vi "MEASURE_hysteresis_multiple_gate_Raman_single 2450 - set voltage - revised for Philipp.vi"() -> ()   [LabVIEW 2016]
uses:
  C/Program Files/National Instruments/LabVIEW 2016/instr.lib/Keithley 2450/Keithley 2450.lvlib
panel:
  out "top gate voltage":dbl format="%#_13g"
  out "loop run":i32=2
  out "top gate leaking":string="-9.306248E-12\n"
  out "while loop":dbl
  in  "Gate sequence":dbl
  in  "GATE final Value":dbl=6.0
  in  "topgate-off set":dbl=-5.0
  in  "0ff set{T}/no off set[F]":bool
  in  "loop #":i32=2
  in  "GATE STEP(mv)":i32=100
  in  "GATE Low Value (default 0)":dbl
  in  "GATE High Value":dbl=6.0
  in  "Function (0: Volts) 2":u16(ring) items=["Volts", "Current", "Resistance"]
  in  "Source Compaliance":dbl=1.000000000000001e-07
  in  "topgate address":refnum<visa-resource-name>="GPIB0::20::INSTR"
  in  "GATE / SD stablization 3":dbl=0.2 format="%#_13g"
  # "Gate 2450 Setting"
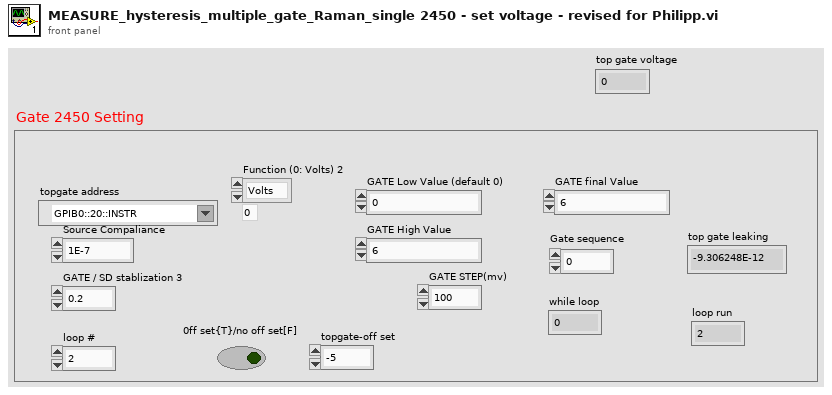
[diagram p1: front panel]
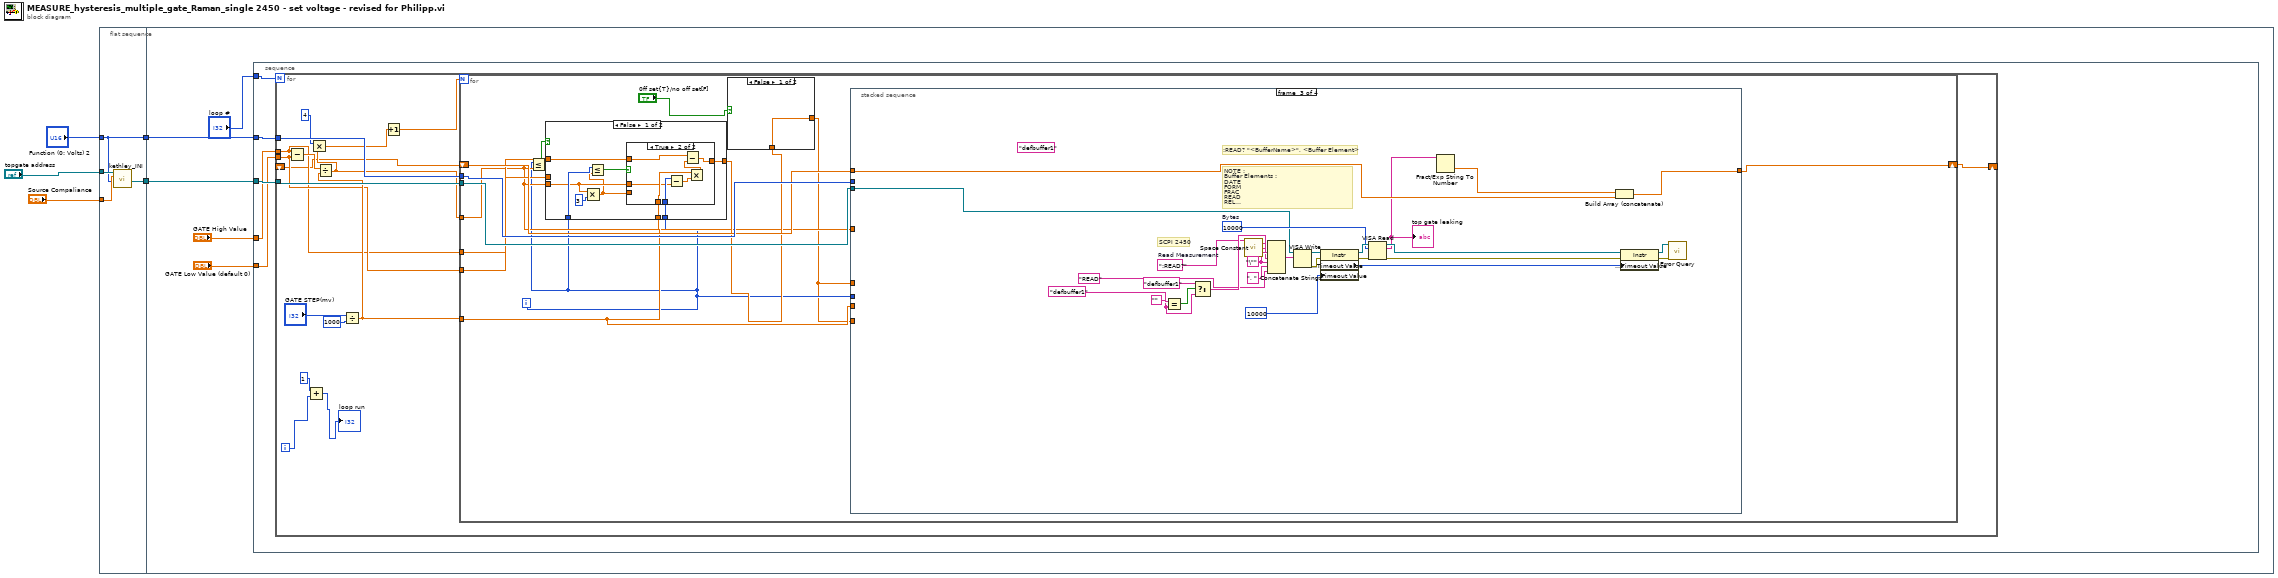
[diagram p0: block diagram]
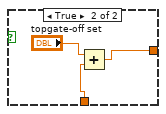
[diagram p2: hidden frame]
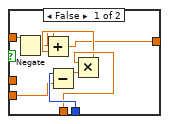
[diagram p3: hidden frame]
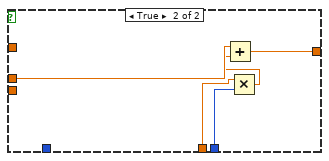
[diagram p4: hidden frame]
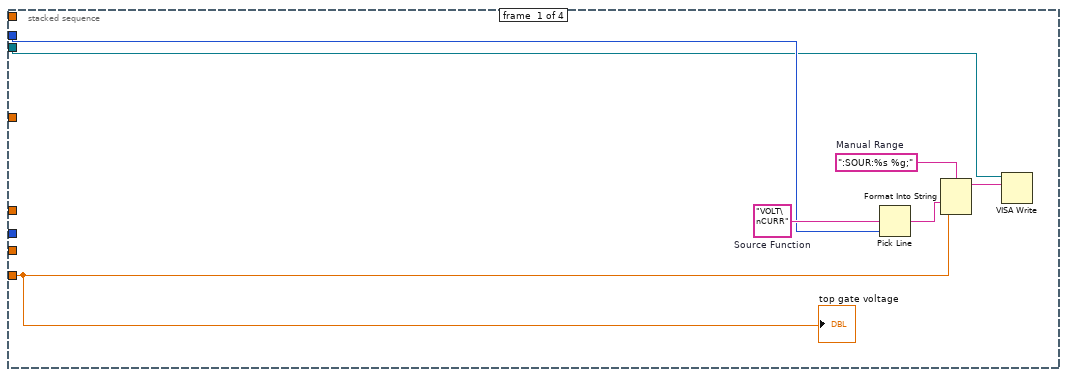
[diagram p5: hidden frame]
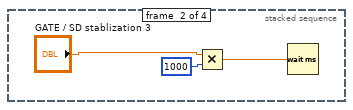
[diagram p6: hidden frame]
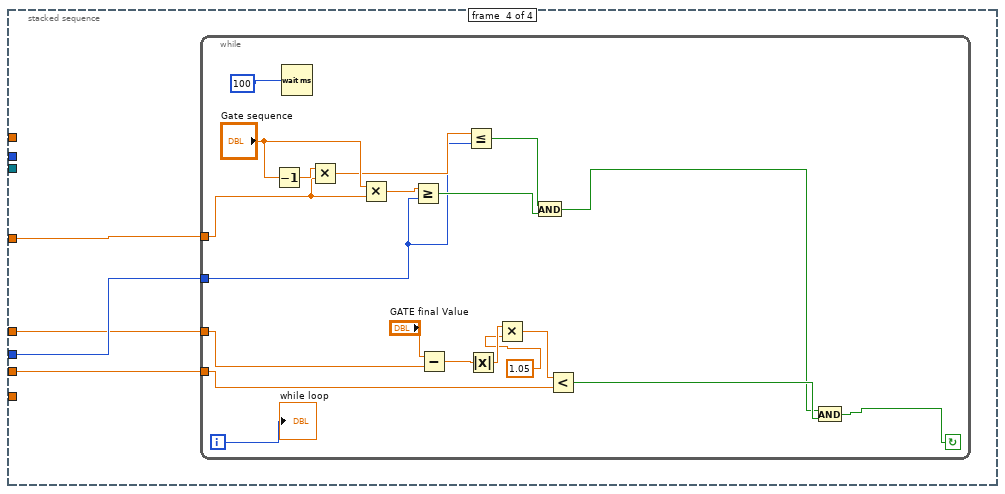
[diagram p7: hidden frame]
diagram:
  n1 = flat-sequence {
    tunnel: "topgate address" -> [w9]
    tunnel: "Source Compaliance" -> [w8]
    tunnel: "Function (0: Volts) 2" -> [w6]
    tunnel: [w7] -> w2
    tunnel: [w6] -> w1
    tunnel: w2 -> [w14]
    tunnel: w1 -> [w13]
    frame #0 {
      n2 = call "kethley_INI.vi"("Function (0: Volts) in"=w6, "Source Compaliance"=w8, "VISA Refnum in"=w9) -> ("VISA resource name out"=w7:refnum<visa-resource-name>)  [unwired: 8 in]
    }
    frame #1 {
      n3 = stacked-sequence {
        tunnel: w14 -> [w18]
        tunnel: w13 -> [w19]
        tunnel: "GATE High Value" -> [w16]
        tunnel: "GATE Low Value (default 0)" -> [w17]
        tunnel: "loop #" -> [w15]
        frame #0 {
          n4 = for {
            N: w15 -> [_]
            tunnel: w19 -> [w36]
            tunnel: w18 -> [w35]
            tunnel: w17 -> [w29]
            tunnel: w16 -> [w28]
            shift-right: [w24] -> _
            shift-left: _ -> [w23]
            i -> [w21]
            n5 = Subtract(x=w28, y=w29) -> (x-y=w31:dbl)
            n6 = Add(x=1, y=w21) -> (x+y=→"loop run":i32)
            n7 = Divide(x="GATE STEP(mv)", y=1000) -> (x/y=w30:dbl)
            n8 = Divide(x=w31, y=w30) -> (x/y=w27:dbl)
            n9 = Multiply(x=4, y=w27) -> (x*y=w26:dbl)
            n10 = Increment(x=w26) -> (x+1=w25:dbl)
            n11 = for {
              N: w25 -> [_]
              tunnel: w36 -> [w49]
              tunnel: w35 -> [w48]
              tunnel: w30 -> [w40]
              shift-right: [w47] -> w24
              shift-left: w23 -> [w46]
              tunnel: w27 -> [w39]
              tunnel: w29 -> [w44]
              tunnel: w28 -> [w43]
              i -> [w38]
              n12 = Less Or Equal?(x=w38, y=w39) -> (x <= y?=w45:bool)
              n13 = case shown="False" w45 {
                tunnel: w44 -> [_ w82]
                tunnel: w38 -> [w62 w81]
                tunnel: w40 -> [w61 w80]
                tunnel: [w59 w78] -> w41
                tunnel: w43 -> [w60 _]
                tunnel: w39 -> [w55 _]
                tunnel: w38 -> [w58 _]
                frame False {
                  n14 = Multiply(x=w55, y=3) -> (x*y=w54:dbl)
                  n15 = Less Or Equal?(x=w58, y=w54) -> (x <= y?=w56:bool)
                  n16 = case shown="True" w56 {
                    tunnel: w62 -> [w70 w77]
                    tunnel: w61 -> [w68 w75]
                    tunnel: w60 -> [w64 w73]
                    tunnel: [w66 w72] -> w59
                    tunnel: w55 -> [_ w71]
                    tunnel: w54 -> [w63 _]
                    frame False {
                      n17 = Negate(x=w64) -> (-x=w65:dbl)
                      n18 = Subtract(x=w70, y=w63) -> (x-y=w69:dbl)
                      n19 = Multiply(x=w68, y=w69) -> (x*y=w67:dbl)
                      n20 = Add(x=w65, y=w67) -> (x+y=w66:dbl)
                    }
                    frame True {
                      n21 = Subtract(x=w77, y=w71) -> (x-y=w76:dbl)
                      n22 = Multiply(x=w75, y=w76) -> (x*y=w74:dbl)
                      n23 = Subtract(x=w73, y=w74) -> (x-y=w72:dbl)
                    }
                  }
                }
                frame True {
                  n24 = Multiply(x=w80, y=w81) -> (x*y=w79:dbl)
                  n25 = Add(x=w82, y=w79) -> (x+y=w78:dbl)
                }
              }
              n26 = case shown="False" "0ff set{T}/no off set[F]" {
                tunnel: w41 -> [w50 w53]
                tunnel: [w50 w51] -> w37
                frame False {
                }
                frame True {
                  n27 = Add(x="topgate-off set", y=w53) -> (x+y=w51:dbl)
                }
              }
              n28 = stacked-sequence {
                tunnel: w49 -> [w85 _ _ _]
                tunnel: w48 -> [w84 _ w97 _]
                tunnel: w37 -> [w83 _ _ _]
                tunnel: [_ _ w95 _] -> w47
                tunnel: w46 -> [_ _ w96 _]
                tunnel: w40 -> [_ _ _ w121]
                tunnel: w39 -> [_ _ _ w122]
                tunnel: w38 -> [_ _ _ w123]
                tunnel: w37 -> [_ _ _ w120]
                frame #0 {
                  w87 = "VOLT\nCURR"  # Source Function
                  w88 = ":SOUR:%s %g;"  # Manual Range
                  n29 = Pick Line(multi-line string=w87, line index=w85) -> (output string=w86:string)  [unwired: 1 out]
                  n30 = Format Into String(format string=w88, w86, w83) -> (resulting string=w89:string)  [unwired: 2 in, 1 out]
                  n31 = VISA Write(VISA resource name=w84, write buffer=w89) -> ()  [unwired: 1 in, 3 out]
                  "top gate voltage" <- w83
                }
                frame #1 {
                  n32 = Multiply(x="GATE / SD stablization 3", y=1000) -> (x*y=w92:dbl)
                  n33 = Wait (ms)(milliseconds to wait=w92) -> ()  [unwired: 1 out]
                }
                frame #2 {
                  w108 = "defbuffer1" ("Buffer Name (defbuffer1) 2")
                  (unwired) "defbuffer1" ("t")
                  w106 = "\""
                  w103 = ":READ?"  # Read Measurement
                  w112 = u32 10000  # Bytes
                  # "NOTE :\nBuffer Elements :\nDATE\nFORM\nFRAC\nREAD\nREL\nSEC\nSOUR\nSOURFORM\nSOURSTAT\nSOURUNIT\nSTAT\nTIME\nTsT\nUNIT"
                  # ":READ? \"<BufferName>\", <Buffer Element>"
                  # "SCPI 2450"
                  n34 = Equal?(x="", y=w108) -> (x = y?=w109:bool)
                  n35 = Select(t="defbuffer1", s=w109, f=w108) -> (s? t:f=w105:string)
                  n36 = call <vilib>:"Space Constant.vi"() -> ("String"=w104:string)
                  n37 = Concatenate Strings(w103, w104, w106, w105, w106, ", " ("string"), "READ" ("Buffer Elements 2")) -> (w119:string)
                  n38 = VISA Write(VISA resource name=w97, write buffer=w119) -> (VISA resource name out=w111:refnum<visa-resource-name>, error out=w118:errorcluster)  [unwired: 1 in, 1 out]
                  n39 = property class="Instr"(reference=w111, error in=w118, "General Settings:Timeout Value"=10000 ("Timeout (10000 ms) 2")) -> (reference out=w117:refnum<visa-resource-name>, error out=w116:errorcluster, "General Settings:Timeout Value"=w113:u32)
                  n40 = VISA Read(VISA resource name=w117, byte count=w112, error in (no error)=w116) -> (VISA resource name out=w115:refnum<visa-resource-name>, read buffer=w93:string, error out=w114:errorcluster)  [unwired: 1 out]
                  "top gate leaking" <- w93
                  n41 = Fract/Exp String To Number(string=w93) -> (number=w94:dbl)  [unwired: 3 in, 1 out]
                  n42 = Build Array (concatenate)(w94, w96) -> (w95:dbl[])
                  n43 = property class="Instr"(reference=w115, error in=w114, "General Settings:Timeout Value"=w113) -> (reference out=w101:refnum<visa-resource-name>, error out=w100:errorcluster)
                  n44 = call "Error Query.vi"("error in (no error)"=w100, "VISA resource name"=w101) -> ()  [unwired: 10 out]
                }
                frame #3 {
                  n45 = while {
                    tunnel: w123 -> [w129]
                    tunnel: w122 -> [w133]
                    tunnel: w121 -> [w138]
                    tunnel: w120 -> [w136]
                    i -> [w143]
                    stop <- w141 continue-if-true
                    n46 = Decrement(x="Gate sequence") -> (x-1=w134:dbl)
                    n47 = Wait (ms)(milliseconds to wait=100) -> ()  [unwired: 1 out]
                    n48 = Multiply(x=w134, y=w133) -> (x*y=w130:dbl)
                    n49 = Multiply(x="Gate sequence", y=w133) -> (x*y=w132:dbl)
                    n50 = Greater Or Equal?(x=w132, y=w129) -> (x >= y?=w131:bool)
                    n51 = Subtract(x="GATE final Value", y=w136) -> (x-y=w139:dbl)
                    n52 = Less Or Equal?(x=w130, y=w129) -> (x <= y?=w128:bool)
                    n53 = Absolute Value(x=w139) -> (abs(x)=w126:dbl)
                    n54 = Multiply(x=w126, y=1.05) -> (x*y=w125:dbl)
                    n55 = And(x=w128, y=w131) -> (x .and. y?=w127:bool)
                    n56 = Less?(x=w125, y=w138) -> (x < y?=w137:bool)
                    n57 = And(x=w127, y=w137) -> (x .and. y?=w141:bool)
                    "while loop" <- w143
                  }
                }
              }
            }
          }
        }
      }
    }
  }
